vi "Test Synchronize DAQ.vi"() -> ()   [LabVIEW 2019, in "Instrument.Lockin.lvlib" / "Instrument.DAQ.lvclass"]
uses:
  Instrument.DAQ.lvclass
  <vilib>/measure/NI_MABase.lvlib
  <vilib>/DAQmx/write.llb/DAQmx Write (Analog 1D Wfm NChan NSamp).vi
  <resource>/objmgr/daqmx.rc
  <vilib>/DAQmx/read.llb/DAQmx Read (Analog 1D Wfm NChan NSamp).vi
  Typedefs/DAQ.Config.AI.Coupling--enum.ctl
  Typedefs/DAQ.Config.AI.Range--enum.ctl
  Typedefs/DAQ.Type--enum.ctl
  Typedefs/DAQ.Config.AI--Cluster.ctl
  Typedefs/DAQ.Config.AO.Range--enum.ctl
  Typedefs/DAQ.Config.AO--Cluster.ctl
  Typedefs/DAQ.Sampling.Sample Mode--Ring.ctl
  Typedefs/DAQ.Sampling.Sampling--Cluster.ctl
panel:
  in  "frequency":dbl=10.0 format="%0.2p"
  out "Waveform Graph":dbl[][](graph)
  in  "stop":bool
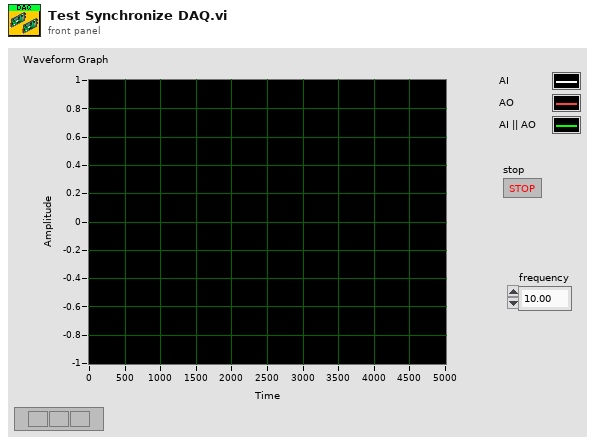
[diagram p1: front panel]
types:
  T1 = typedef "Instrument.Lockin.lvlib/Instrument.DAQ.lvclass/DAQ.Sampling.Sampling--Cluster.ctl" = cluster{"Fs":dbl, "#s":i32}
  T2 = typedef "Instrument.Lockin.lvlib/Instrument.DAQ.lvclass/DAQ.Sampling.Sample Mode--Ring.ctl" = i32
  T3 = typedef "Instrument.Lockin.lvlib/Instrument.DAQ.lvclass/DAQ.Config.AO--Cluster.ctl" = cluster{"Channels":tag, "Range":T4, "output terminal configuration":i32, "Type":T5}
  T4 = typedef "Instrument.Lockin.lvlib/Instrument.DAQ.lvclass/DAQ.Config.AO.Range--enum.ctl" = enum16{"±0.1", "±1.0", "±10.0", ""}
  T5 = typedef "Instrument.Lockin.lvlib/Instrument.DAQ.lvclass/DAQ.Type--enum.ctl" = enum16{"None", "USB-4431", "PXI-446x"}
  T6 = typedef "Instrument.Lockin.lvlib/Instrument.DAQ.lvclass/DAQ.Config.AI--Cluster.ctl" = cluster{"Channels":tag, "Coupling":T7, "Range":T8, "input terminal configuration":i32, "Type":T5}
  T7 = typedef "Instrument.Lockin.lvlib/Instrument.DAQ.lvclass/DAQ.Config.AI.Coupling--enum.ctl" = u16
  T8 = typedef "Instrument.Lockin.lvlib/Instrument.DAQ.lvclass/DAQ.Config.AI.Range--enum.ctl" = enum16{"±0.316", "±1.00", "±3.16", "±10.0", "±31.6", "±42.4", ""}
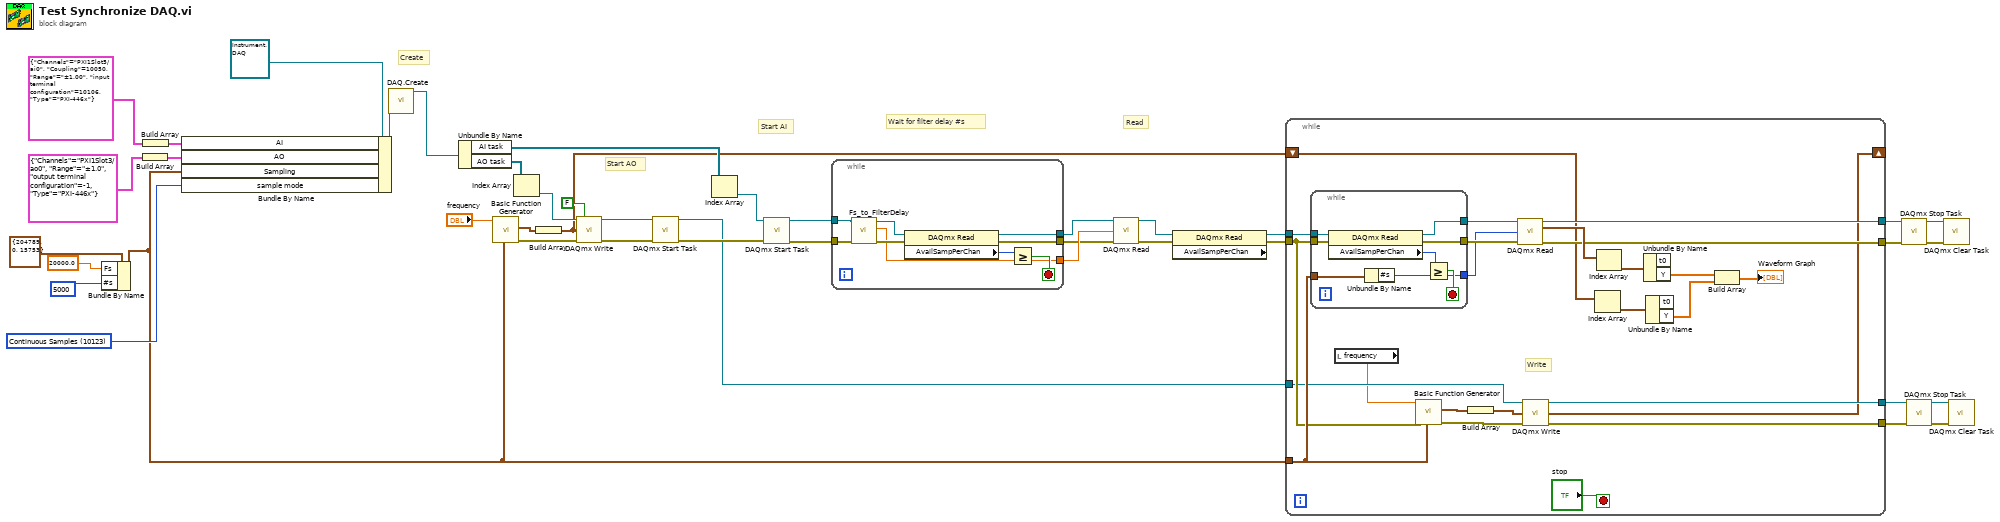
[diagram p0: block diagram]
diagram:
  w7 = T2 10123 items=["Finite Samples"=10178, "Continuous Samples"=10123] ("Configuration.DAQ.Sampling.Sample Mode")
  # "Read"
  # "Wait for filter delay #s"
  # "Start AI"
  # "Start AO"
  # "Create"
  n1 = Bundle By Name(cluster=T1 {"Fs"=204789.0, "#s"=15753} ("Configuration.DAQ.Sampling.Sampling"), "Fs"=20000.0, "#s"=5000) -> (w3:T1)
  n2 = Build Array(T3 {"Channels"="PXI1Slot3/ao0", "Range"=enum."±1.0", "output terminal configuration"=-1, "Type"=enum."PXI-446x"} ("AO.config")) -> (w18:T3[])
  n3 = Build Array(T6 {"Channels"="PXI1Slot5/ai0", "Coupling"=10050, "Range"=enum."±1.00", "input terminal configuration"=10106, "Type"=enum."PXI-446x"} ("AI.Config")) -> (w19:T6[])
  n4 = Bundle By Name(cluster=refnum<class "Instrument.DAQ.lvclass"> refnum ("Instrument.DAQ"), "AI"=w19, "AO"=w18, "Sampling"=w3, "sample mode"=w7) -> (w36:refnum<class "Instrument.DAQ.lvclass">)
  n5 = call "DAQ.Create.vi"("Instrument.DAQ"=w36) -> ("Instrument.DAQ"=w42:refnum<class "Instrument.DAQ.lvclass">)  [unwired: 9 in, 1 out]
  n6 = Unbundle By Name(w42) -> ("AI task"=w31:refnum<k21>[], "AO task"=w40:refnum<k21>[])
  n7 = call <vilib>:"Basic Function Generator.vi"("sampling info"=w3, "frequency"="frequency") -> ("error out"=w33:errorcluster, "signal out"=w38:waveform(dbl))  [unwired: 7 in, 1 out]
  n8 = Index Array(array=w40) -> (element=w39:refnum<k21>)  [unwired: 1 in]
  n9 = Build Array(w38) -> (w2:waveform(dbl)[])
  n10 = call-poly <vilib>:"DAQmx Write.vi"("task/channels in"=w39, "auto start"=FALSE, "data"=w2, "error in"=w33) -> ("task out"=w35:refnum<k21>, "error out"=w34:errorcluster)  [unwired: 9 in, 1 out]
  n11 = call <vilib>:"DAQmx Start Task.vi"("task/channels in"=w35, "error in"=w34) -> ("task out"=w16:refnum<k21>, "error out"=w25:errorcluster)  [unwired: 12 in]
  n12 = Index Array(array=w31) -> (element=w32:refnum<k21>)  [unwired: 1 in]
  n13 = call <vilib>:"DAQmx Start Task.vi"("task/channels in"=w32, "error in"=w25) -> ("task out"=w29:refnum<k21>, "error out"=w30:errorcluster)  [unwired: 12 in]
  n14 = while {
    tunnel: w30 -> [w47]
    tunnel: w29 -> [w43]
    tunnel: [w49] -> w26
    tunnel: [w44] -> w28
    tunnel: [w48] -> w27
    stop <- w50 stop-if-true
    n15 = call "Fs_to_FilterDelay.vi"("error in (no error)"=w47, "Refnum in"=w43) -> ("error out"=w45:errorcluster, "Total Filter Delay (samples)"=w44:dbl, "Refnum out"=w46:refnum<k21>)  [unwired: 7 in]
    n16 = property class="DAQmx Read"(reference=w46, error in=w45) -> (reference out=w49:refnum<k21>, error out=w48:errorcluster, "AvailSampPerChan"=w51:u32)
    n17 = Greater Or Equal?(x=w51, y=w44) -> (x >= y?=w50:bool)
  }
  n18 = call-poly <vilib>:"DAQmx Read.vi"("task/channels in"=w26, "number of samples per channel"=w28, "error in"=w27) -> ("task out"=w24:refnum<k21>, "error out"=w23:errorcluster)  [unwired: 10 in, 1 out]
  n19 = property class="DAQmx Read" props=["AvailSampPerChan"](reference=w24, error in=w23) -> (reference out=w22:refnum<k21>, error out=w21:errorcluster)  [unwired: 1 out]
  n20 = while {
    tunnel: w22 -> [w74]
    tunnel: w21 -> [w69]
    tunnel: w16 -> [w60]
    tunnel: w3 -> [w70]
    tunnel: [w59] -> w15
    tunnel: [w58] -> w14
    tunnel: [w57] -> w9
    tunnel: [w56] -> w8
    shift-right: [w54] -> _
    shift-left: w2 -> [w53]
    stop <- "stop" stop-if-true
    # "Write"
    n21 = while {
      tunnel: w74 -> [w82]
      tunnel: w69 -> [w81]
      tunnel: [w80] -> w73
      tunnel: [w79] -> w72
      tunnel: w70 -> [w76]
      tunnel: [w75] -> w55
      stop <- w77 stop-if-true
      n22 = property class="DAQmx Read"(reference=w82, error in=w81) -> (reference out=w80:refnum<k21>, error out=w79:errorcluster, "AvailSampPerChan"=w78:u32)
      n23 = Unbundle By Name(w76) -> ("#s"=w75:i32)
      n24 = Greater Or Equal?(x=w78, y=w75) -> (x >= y?=w77:bool)
    }
    n25 = local read "frequency"() -> (w52:dbl)
    n26 = call <vilib>:"Basic Function Generator.vi"("sampling info"=w70, "error in (no error)"=w69, "frequency"=w52) -> ("error out"=w61:errorcluster, "signal out"=w71:waveform(dbl))  [unwired: 6 in, 1 out]
    n27 = Build Array(w71) -> (w54:waveform(dbl)[])
    n28 = call-poly <vilib>:"DAQmx Read.vi"("task/channels in"=w73, "number of samples per channel"=w55, "error in"=w72) -> ("task out"=w59:refnum<k21>, "data"=w64:waveform(dbl)[], "error out"=w58:errorcluster)  [unwired: 10 in]
    n29 = call-poly <vilib>:"DAQmx Write.vi"("task/channels in"=w60, "data"=w54, "error in"=w61) -> ("task out"=w57:refnum<k21>, "error out"=w56:errorcluster)  [unwired: 10 in, 1 out]
    n30 = Index Array(array=w53) -> (element=w66:waveform(dbl))  [unwired: 1 in]
    n31 = Index Array(array=w64) -> (element=w65:waveform(dbl))  [unwired: 1 in]
    n32 = Unbundle By Name(w65) -> ("Y"=w63:dbl[])  [unwired: 1 out]
    n33 = Unbundle By Name(w66) -> ("Y"=w62:dbl[])  [unwired: 1 out]
    n34 = Build Array(w63, w62) -> (→"Waveform Graph":dbl[][])
  }
  n35 = call <vilib>:"DAQmx Stop Task.vi"("task/channels in"=w15, "error in"=w14) -> ("task out"=w12:refnum<k21>, "error out"=w13:errorcluster)  [unwired: 12 in]
  n36 = call <vilib>:"DAQmx Stop Task.vi"("task/channels in"=w9, "error in"=w8) -> ("task out"=w11:refnum<k21>, "error out"=w10:errorcluster)  [unwired: 12 in]
  n37 = call <vilib>:"DAQmx Clear Task.vi"("task in"=w12, "error in"=w13) -> ()  [unwired: 13 in, 1 out]
  n38 = call <vilib>:"DAQmx Clear Task.vi"("task in"=w11, "error in"=w10) -> ()  [unwired: 13 in, 1 out]
